vi "sv_Number of Chirp Samples Left.vi"(0 "frequency slope":dbl, 1 "initial states":T1={"frequency [Hz]"=20.0, "phase [rad]"=0.0, "elapsed time [s]"=0.0} {"elapsed time [s]" format="%.2f"; "phase [rad]" format="%.2f"; "frequency [Hz]" format="%.2f"}, 7 "frequency range":cluster{"start (Hz)":dbl, "stop (Hz)":dbl}={"start (Hz)"=20.0, "stop (Hz)"=20000.0} {"stop (Hz)" format="%.2f"; "start (Hz)" format="%.2f"}, 11 "error in (no error)":errorcluster, 13 "frequency spacing":enum16{"Linear", "Logarithmic"}(ring)) -> (3 "initial states out":T1={"frequency [Hz]"=20.0, "phase [rad]"=0.0, "elapsed time [s]"=0.0} {"elapsed time [s]" format="%.2f"; "phase [rad]" format="%.2f"; "frequency [Hz]" format="%.2f"}, 4 "# of samples left":i32, 15 "error out":errorcluster)   [LabVIEW 2017, in "SoundVib_Generation.lvlib"]
uses:
  <vilib>/addons/_NISVFA/_Generation/SoundVib_Generation.lvlib
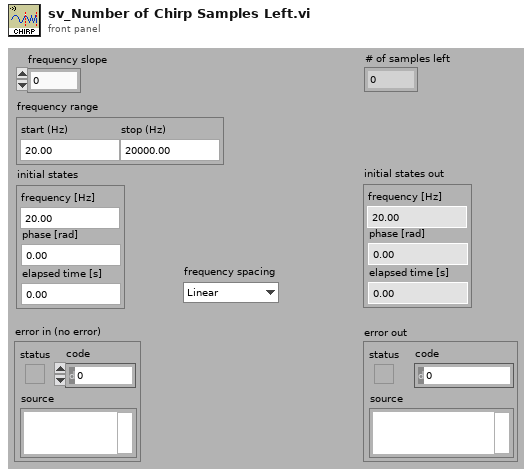
[diagram p1: front panel]
types:
  T1 = cluster{"frequency [Hz]":dbl, "phase [rad]":dbl, "elapsed time [s]":dbl}
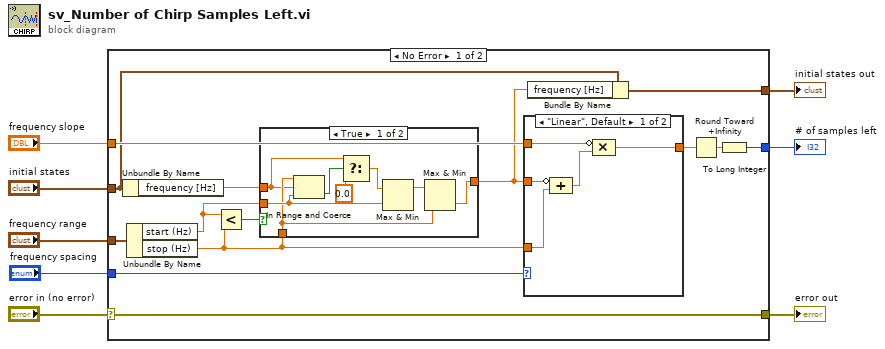
[diagram p0: block diagram]
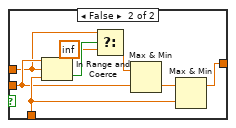
[diagram p2: hidden frame]
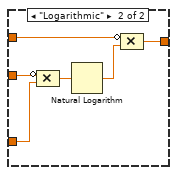
[diagram p3: hidden frame]
diagram:
  n1 = case shown="No Error" "error in (no error)" {
    selector: "error in (no error)" -> [w17 w51]
    tunnel: "frequency slope" -> [w21 _]
    tunnel: "initial states" -> [w16 w50]
    tunnel: "frequency range" -> [w22 _]
    tunnel: [w18 _] -> w4
    tunnel: [w17 w51] -> w3
    tunnel: [w15 w50] -> w2
    tunnel: "frequency spacing" -> [w14 _]
    frame No Error {
      n2 = Unbundle By Name(w16) -> ("frequency [Hz]"=w12:dbl)
      n3 = Unbundle By Name(w22) -> ("start (Hz)"=w11:dbl, "stop (Hz)"=w10:dbl)
      n4 = Less?(x=w11, y=w10) -> (x < y?=w13:bool)
      n5 = case shown="True" w13 {
        tunnel: w12 -> [w25 w33]
        tunnel: w11 -> [w28 w35]
        tunnel: w10 -> [w27 w36]
        tunnel: [w29 w37] -> w9
        frame True {
          n6 = In Range and Coerce(upper limit=w27, x=w25, lower limit=w28) -> (In Range?=w26:bool)  [unwired: 1 out]
          n7 = Select(t=w25, s=w26, f=0.0) -> (s? t:f=w23:dbl)
          n8 = Max & Min(x=w23, y=w28) -> (max(x,y)=w30:dbl)  [unwired: 1 out]
          n9 = Max & Min(x=w30, y=w27) -> (min(x,y)=w29:dbl)  [unwired: 1 out]
        }
        frame False {
          n10 = In Range and Coerce(upper limit=w35, x=w33, lower limit=w36) -> (In Range?=w34:bool)  [unwired: 1 out]
          n11 = Select(t=w33, s=w34, f=inf) -> (s? t:f=w31:dbl)
          n12 = Max & Min(x=w31, y=w35) -> (min(x,y)=w38:dbl)  [unwired: 1 out]
          n13 = Max & Min(x=w38, y=w36) -> (max(x,y)=w37:dbl)  [unwired: 1 out]
        }
      }
      n14 = case shown="\"Linear\", Default" w14 {
        tunnel: w10 -> [w42 w48]
        tunnel: w9 -> [w43 w49]
        tunnel: w21 -> [w40 w45]
        tunnel: [w39 w44] -> w20
        frame "Linear", Default {
          n15 = Compound Arithmetic op=ADD(invert w43, w42) -> (w41:dbl)
          n16 = Compound Arithmetic op=MULTIPLY(invert w40, w41) -> (w39:dbl)
        }
        frame "Logarithmic" {
          n17 = Compound Arithmetic op=MULTIPLY(invert w49, w48) -> (w47:dbl)
          n18 = Natural Logarithm(1:w47) -> (0:w46:dbl)
          n19 = Compound Arithmetic op=MULTIPLY(invert w45, w46) -> (w44:dbl)
        }
      }
      n20 = Bundle By Name(cluster=w16, "frequency [Hz]"=w9) -> (w15:T1)
      n21 = Round Toward +Infinity(x=w20) -> (ceil(x): smallest int >= x=w19:dbl)
      n22 = To Long Integer(number=w19) -> (32bit integer=w18:i32)
    }
    frame Error {
    }
  }
  "# of samples left" <- w4
  "error out" <- w3
  "initial states out" <- w2
